vi "Initialize Manager Tab.vi"(8 "error in (no error)":errorcluster, 11 "CIF Manager UI Tab":refnum<vi>) -> (0 "error out":errorcluster)   [LabVIEW 2021, in "CIF_UI.lvclass"]
uses:
  CIF_UI.lvclass
  Typedef/CIF_Manager_UI_Tab.ctl
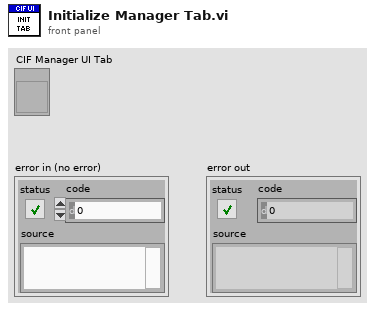
[diagram p1: front panel]
types:
  T1 = typedef "CIF_Manager_UI_Tab.ctl" = enum32{"System Management", "Channels", "Monitoring and Errors", "Plugin", "Plugin2", "Plugin3", "Plugin4", "Plugin5", "Plugin6", "Plugin7", "Plugin8", "Plugin9", "Plugin10"}
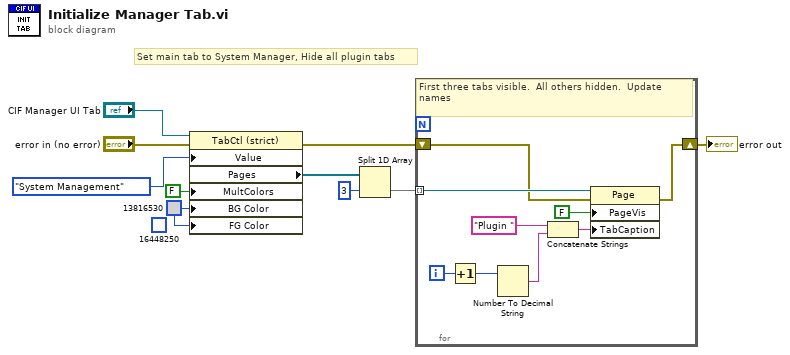
[diagram p0: block diagram]
diagram:
  (unwired) u32 16448250 ("Colors:FG Color")
  w1 = u32 13816530 ("Colors:BG Color")
  # "Set main tab to System Manager, Hide all plugin tabs"
  n1 = property on="Property Node" class="TabCtl (strict)"(reference="CIF Manager UI Tab", error in="error in (no error)", "Value"=CIF_Manager_UI_Tab."System Management", "MultColors"=FALSE ("Allow Multiple Colors"), "BG Color"=w1, "FG Color"=w1) -> (error out=w7:errorcluster, "Pages"=w5:refnum<vi>[])  [unwired: 1 out]
  n2 = Split 1D Array(array=w5, index=3) -> (second subarray=w3:refnum<vi>[])  [unwired: 1 out]
  n3 = for {
    tunnel: w3 -> [w19] mode=indexing
    shift-right: [w17] -> w6
    shift-left: w7 -> [w18]
    i -> [w15]
    # "First three tabs visible.  All others hidden.  Update names"
    n4 = Increment(x=w15) -> (x+1=w14:i32)
    n5 = Number To Decimal String(number=w14) -> (decimal integer string=w13:string)  [unwired: 1 in]
    n6 = Concatenate Strings("Plugin " ("string"), w13) -> (w11:string)
    n7 = property on="Property Node" class="Page"(reference=w19, error in=w18, "PageVis"=FALSE ("Page Visible"), "TabCaption"=w11) -> (error out=w17:errorcluster)  [unwired: 1 out]
  }
  "error out" <- w6
